vi "Charts and Graphs.vi"() -> ()   [LabVIEW 2014]
panel:
  out "Graph":dbl[](graph)
  out "Chart":dbl(graph)
  # "CHARTS AND GRAPHS"
  # "Chart (Updated Instantly)"
  # "Graph(Updated every 11 pts)"
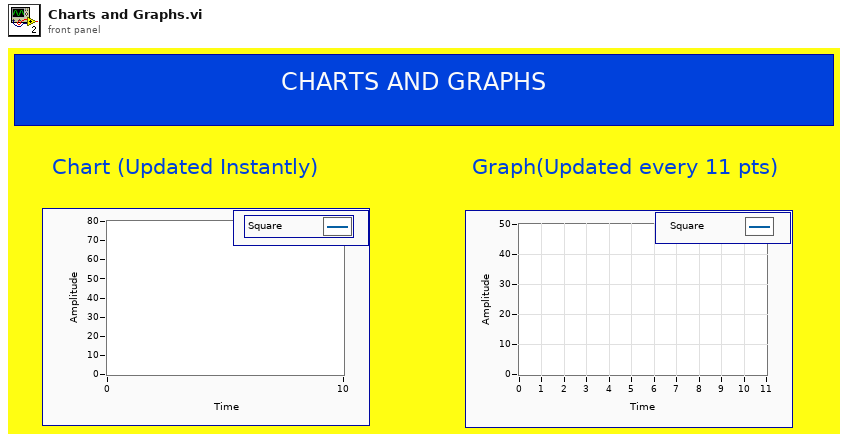
[diagram p1: front panel]
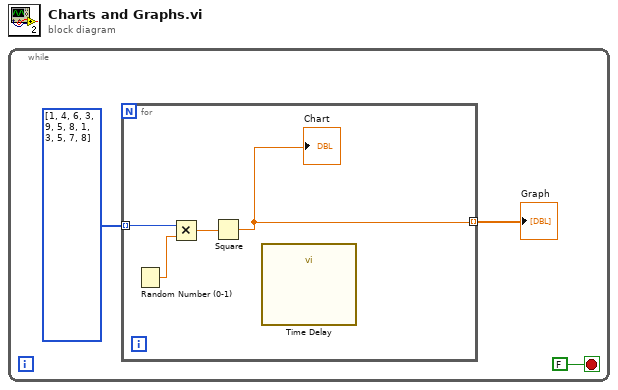
[diagram p0: block diagram]
diagram:
  n1 = while {
    stop <- FALSE stop-if-true
    n2 = for {
      tunnel: i32[] [1, 4, 6, 3, 9, 5, 8, 1, 3, 5, 7, 8] -> [w7] mode=indexing
      tunnel: [w4] -> w1 mode=indexing
      n3 = Random Number (0-1)() -> (number: 0 to 1=w6:dbl)
      n4 = Multiply(x=w7, y=w6) -> (x*y=w5:dbl)
      n5 = Square(x=w5) -> (x^2=w4:dbl)
      "Chart" <- w4
      n6 = call "Time Delay"() -> ()  [unwired: 11 in, 1 out]
    }
    "Graph" <- w1
  }
